vi "GetExplicitMessage.vi"(8 "error in (no error)":errorcluster, 10 "Motor Controller Parameter":T1, 11 ".NET Refnum in":refnum<k24>) -> (0 "error out":errorcluster, 1 "GetAttributeSingle":u8[](array[numeric]), 2 "size":i32, 3 ".NET Refnum out":refnum<k24>, 4 "Data (U32)":u32)   [LabVIEW 2022 SP3]
uses:
  C:/projects/Digilens_IPLC2/Classes/Motor Controller/EEIP.dll
  EEIP.dll
  Typedefs/Motor Controller Parameter-Get.ctl
  Motor Controller.lvclass
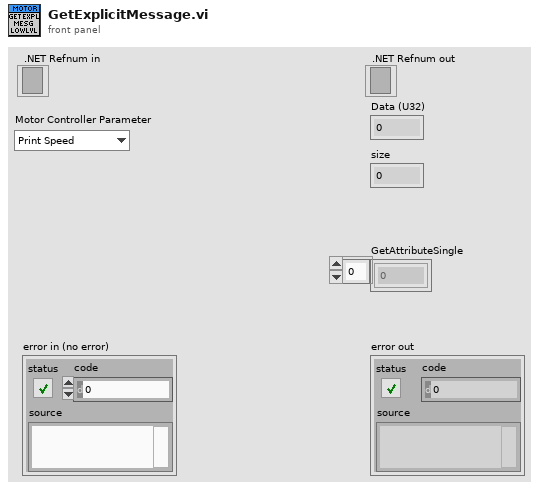
[diagram p1: front panel]
types:
  T1 = typedef "Motor Controller.lvclass/Motor Controller Parameter-Get.ctl" = enum16{"Print Speed", "Jog Speed", "PR Path", "Servo Enabled?", "AlarmCodes"}
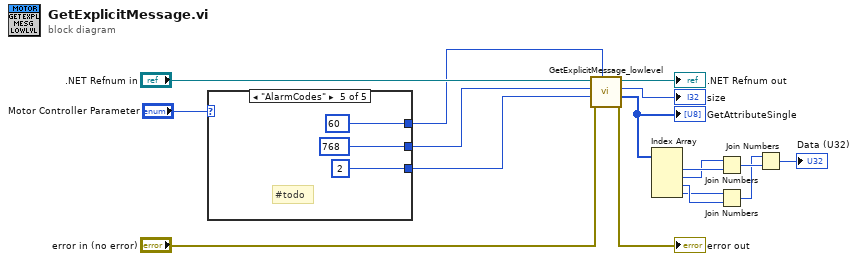
[diagram p0: block diagram]
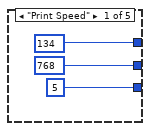
[diagram p2: hidden frame]
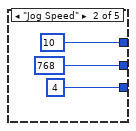
[diagram p3: hidden frame]
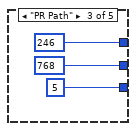
[diagram p4: hidden frame]
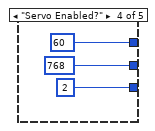
[diagram p5: hidden frame]
diagram:
  n1 = case shown="\"AlarmCodes\"" "Motor Controller Parameter" {
    tunnel: [134 ("Attribute") 10 ("Attribute") 246 ("Attribute") 60 ("Attribute") 60 ("Attribute")] -> w11
    tunnel: [768 ("Class") 768 ("Class") 768 ("Class") 768 ("Class") 768 ("Class")] -> w10
    tunnel: [u32 5 ("assembly instance ID") u32 4 ("assembly instance ID") u32 5 ("assembly instance ID") u32 2 ("assembly instance ID") u32 2 ("assembly instance ID")] -> w9
    frame "Print Speed" {
    }
    frame "Jog Speed" {
    }
    frame "PR Path" {
    }
    frame "Servo Enabled?" {
    }
    frame "AlarmCodes" {
      # "#todo"
    }
  }
  n2 = call "GetExplicitMessage_lowlevel.vi"("Attribute"=w11, "error in (no error)"="error in (no error)", "assembly instance ID"=w9, "Class"=w10, ".NET Refnum in"=".NET Refnum in") -> ("error out"=→"error out":errorcluster, "GetAttributeSingle"=w2:u8[], "Numeric"=→"size":i32, ".NET Refnum out"=→".NET Refnum out":refnum<k24>)  [unwired: 3 in]
  "GetAttributeSingle" <- w2
  n3 = Index Array(array=w2) -> (element #1=w8:u8, element #2=w7:u8, element #3=w6:u8, element #4=w5:u8)  [unwired: 4 in]
  n4 = Join Numbers(hi=w7, lo=w8) -> ((hi.lo)=w4:u16)
  n5 = Join Numbers(hi=w5, lo=w6) -> ((hi.lo)=w3:u16)
  n6 = Join Numbers(hi=w3, lo=w4) -> ((hi.lo)=→"Data (U32)":u32)
